vi "Init-RotateFileHandler.vi"(4 "RotatorArgs":T1={"MaxSize_KB"=10024, "Compress"=FALSE, "MaxBackups"=5}, 5 "Formatter.lvclass":refnum<class "Formatter.lvclass">, 6 "Flush Timeout_s (5 s)":dbl=5.0 format="%#_13g", 7 "Filepath":path, 8 "error in (no error)":errorcluster, 9 "Level":T2, 10 "Name":string, 11 "FileHandler in":refnum<class "RotateFileHandler.lvclass">) -> (0 "error out":errorcluster, 3 "FileHandler out":refnum<class "RotateFileHandler.lvclass">)   [LabVIEW 2024, in "RotateFileHandler.lvclass"]
uses:
  RotateFileHandler.lvclass
  <vilib>/Hampel Software Engineering/HSE Logger/Formatter/Formatter.lvclass
  <vilib>/Hampel Software Engineering/HSE Logger/LogLevel.ctl
  LogRotation/Args.ctl
  RotateFileHandler.lvclass/RotateFileHandler.ctl
  LogRotation/LogRotationHandler.lvclass
  <vilib>/Hampel Software Engineering/HSE Logger/hse-logger.lvlib
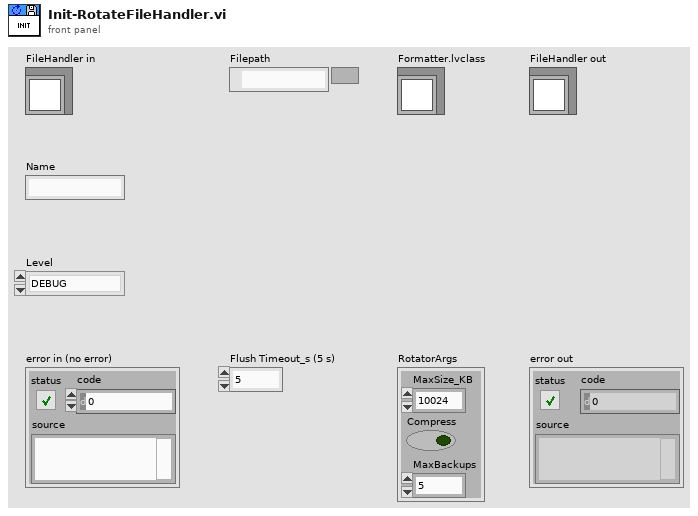
[diagram p1: front panel]
types:
  T1 = typedef "LogRotationHandler.lvclass/Args.ctl" = cluster{"MaxSize_KB":i32, "Compress":bool, "MaxBackups":i32}
  T2 = typedef "hse-logger.lvlib/LogLevel.ctl" = enum16{"DEBUG", "INFO", "WARNING", "ERROR", "CRITICAL"}
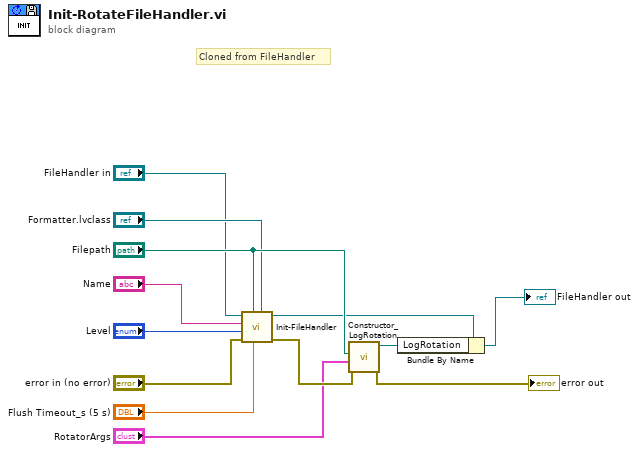
[diagram p0: block diagram]
diagram:
  # "Cloned from FileHandler"
  n1 = call-dynamic "Init-FileHandler.vi"("Formatter.lvclass"="Formatter.lvclass", "Flush Timeout (5 s)"="Flush Timeout_s (5 s)", "Filepath"="Filepath", "error in"="error in (no error)", "Level"="Level", "Name"="Name", "FileHandler"="FileHandler in") -> ("error out"=w12:errorcluster, "FileHandler out"=w8:refnum<class "RotateFileHandler.lvclass">)  [unwired: 3 in]
  n2 = call "Constructor_LogRotation.vi"("error in (no error)"=w12, "Args"="RotatorArgs", "Filepath"="Filepath") -> ("error out"=→"error out":errorcluster, "LogRotationHandler out"=w10:refnum<class "LogRotationHandler.lvclass">)  [unwired: 7 in]
  n3 = Bundle By Name(cluster=w8, "LogRotation"=w10) -> (→"FileHandler out":refnum<class "RotateFileHandler.lvclass">)
